vi "ROI grp-Prevent invalid ROI numbers entry.vi"(8 "error in (no error)":errorcluster, 10 "NewVal in":string[][](array[string]), 11 "OldVal":string[][](array[string])) -> (0 "error out":errorcluster, 2 "Val out":string[][](array[string]), 3 "Discard":bool)   [LabVIEW 2017]
uses:
  <vilib>/Utility/miscctls.llb/LVRowAndColumnTypeDef.ctl
  Typedefs/Get-Set-Clear Control.ctl
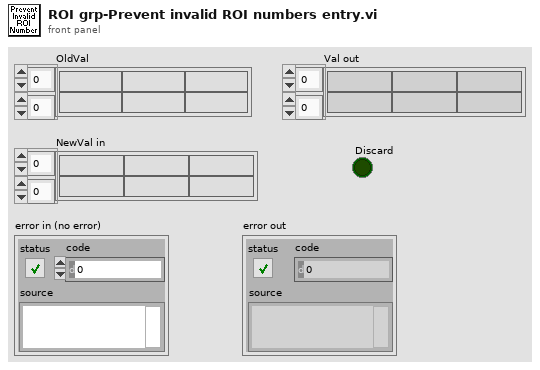
[diagram p1: front panel]
types:
  T1 = typedef "LVRowAndColumnTypeDef.ctl" = cluster{"Row":i32, "Column":i32}
  T2 = typedef "Get-Set-Clear Control.ctl" = enum16{"Get", "Set", "Clear"}
  T3 = typedef "ROI selector array-ROI vis.ctl" = T4[]
  T4 = typedef "Interface-ROI selection cluster.ctl" = cluster{"ROI number":i32, "ROI ID":T5, "Visibility":bool}
  T5 = typedef "ROI ID Enum.ctl" = enum16{"Point", "MiniScan", "Comp. MiniScan", "Rectangle", "Comp. volume", "Arb. plane point"}
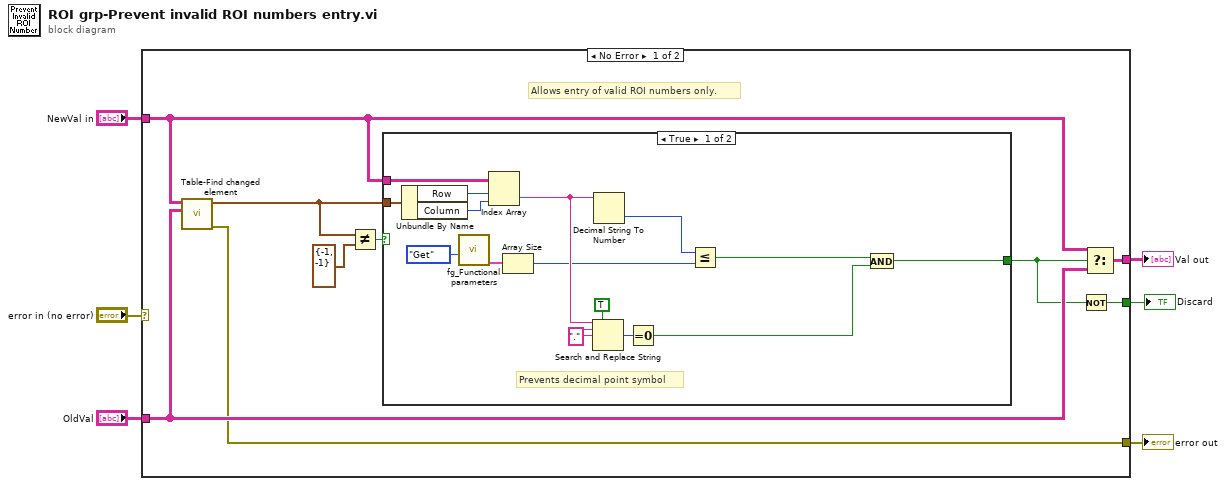
[diagram p0: block diagram]
diagram:
  n1 = case shown="No Error" "error in (no error)" {
    selector: "error in (no error)" -> [_ w32]
    tunnel: [w15 w31] -> w6
    tunnel: "NewVal in" -> [w8 w31]
    tunnel: "OldVal" -> [w14 _]
    tunnel: [w13 w32] -> w3
    tunnel: [w11 _] -> w1
    frame No Error {
      # "Allows entry of valid ROI numbers only."
      n2 = call <userlib>:"Table-Find changed element.vi"("Table 2"=w14, "Table 1"=w8) -> ("error out"=w13:errorcluster, "Index of change"=w7:T1)  [unwired: 8 in]
      n3 = Not Equal?(x=w7, y=T1 {"Row"=-1, "Column"=-1} ("Index of change")) -> (x != y?=w9:bool)
      n4 = case shown="True" w9 {
        tunnel: [w29 _] -> w12
        tunnel: w8 -> [w25 _]
        tunnel: w7 -> [w24 _]
        frame True {
          w21 = "." ("y")
          # "Prevents decimal point symbol"
          n5 = Unbundle By Name(w24) -> ("Row"=w28:i32, "Column"=w27:i32)
          n6 = call "fg_Functional parameters.vi"("Function"=Get-Set-Clear_Control."Get") -> ("[ROI vis]"=w20:T3)  [unwired: 7 in, 3 out]
          n7 = Index Array(array=w25, index (row)=w28, index (col)=w27) -> (element=w26:string)
          n8 = Array Size(array=w20) -> (size(s)=w18:i32)
          n9 = Search and Replace String(replace all?=TRUE ("replace all? (F)"), input string=w26, search string=w21, replace string=w21) -> (number of replacements=w23:i32)  [unwired: 4 in, 3 out]
          n10 = Decimal String To Number(string=w26) -> (number=w17:i32)  [unwired: 2 in, 1 out]
          n11 = Equal To 0?(x=w23) -> (x = 0?=w22:bool)
          n12 = Less Or Equal?(x=w17, y=w18) -> (x <= y?=w16:bool)
          n13 = And(x=w16, y=w22) -> (x .and. y?=w29:bool)
        }
        frame False {
        }
      }
      n14 = Not(x=w12) -> (.not. x?=w11:bool)
      n15 = Select(t=w8, s=w12, f=w14) -> (s? t:f=w15:string[][])
    }
    frame Error {
    }
  }
  "Val out" <- w6
  "error out" <- w3
  "Discard" <- w1
